vi "BRig_dataBlock_nTrial_NFE.vi"() -> (2 "output_nTrial_NFE":i32)   [LabVIEW 2014]
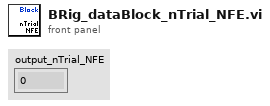
[diagram p1: front panel]
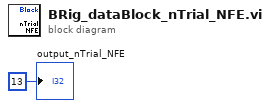
[diagram p0: block diagram]
diagram:
  "output_nTrial_NFE" <- 13 ("output_iBlock")
